vi "ReadFFLoop.vi"(0 "nos":u32=1, 1 "exptus":u32=20000, 2 "freq":u32, 3 "threadp":u32=8, 4 "pixel":u32=2400, 5 "ExtTrig":u8, 7 "releasems":i16) -> (6 "Data Values":u16[][](graph))   [LabVIEW 2015]
uses:
  ESLSCDLL.dll
panel:
  in  "blocktrigger":u8
  in  "clrcnt":u32=8
  in  "zadr":u32=1
  in  "lfkt":i32=1
  in  "lines":u32
  # "lines for  FFTs, or 0 else"
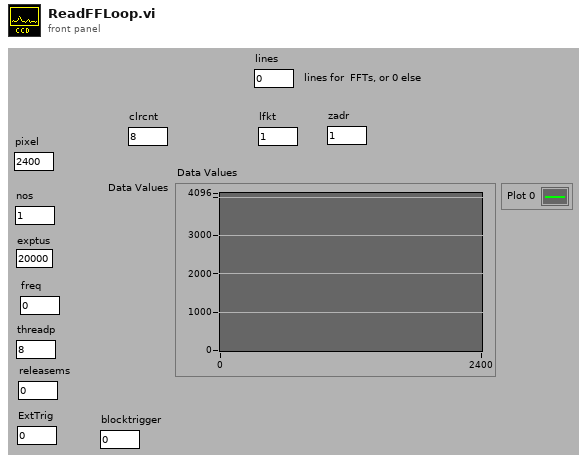
[diagram p1: front panel]
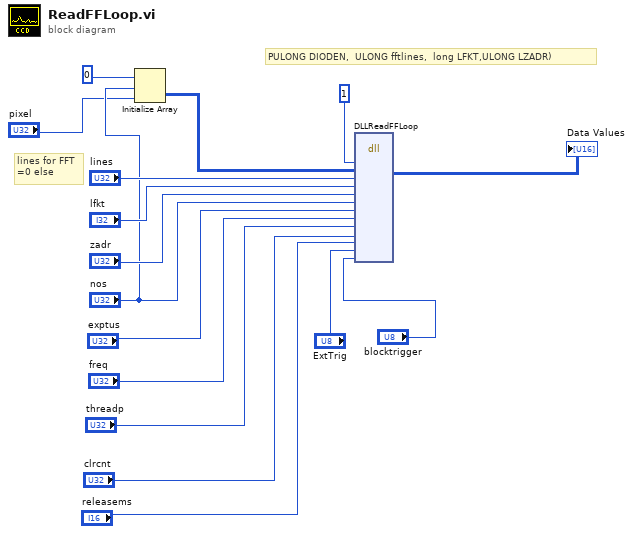
[diagram p0: block diagram]
diagram:
  # "lines for FFT\n=0 else"
  # "PULONG DIODEN, \tULONG fftlines,  long LFKT,ULONG LZADR)"
  n1 = Initialize Array(u32 0, "nos", "pixel") -> (w6:u32[][])
  n2 = dll-call lib="C:/Users/Gerhard/Desktop/GS/lv64/1cam/board.vis/ESLSCDLL.dll" fn="DLLReadFFLoop"("drv"=u32 1, "dioden"=w6, "fftlines"="lines", "fkt"="lfkt", "zadr"="zadr", "nos"="nos", "exptus"="exptus", "freq"="freq", "threadp"="threadp", "clrcnt"="clrcnt", "releasems"="releasems", "exttrig"="ExtTrig", "blocktrigger"="blocktrigger") -> ("dioden"=→"Data Values":u16[][])  [unwired: 16 in, 2 out]
